vi "validate.vi"(8 "error in":errorcluster, 11 "Instrument configuration":refnum<class "Instrument configuration.lvclass">) -> (0 "error out":errorcluster, 3 "Instrument configuration out":refnum<class "Instrument configuration.lvclass">)   [LabVIEW 2025, in "Abstract Engine.lvlib" / "Instrument configuration.lvclass"]
doc: "Provides an interface for performing validation on a given configuration. Any children should define the behavior of this function to ensure that the configuration in memory can be used by the runtime class.Copyright 2017 National Instruments Corporation\n\nLicensed under the Apache License, Version 2.0 (the \"License\"); you may not use this file except in compliance with the License. You may obtain a copy of the License at http://www.apache.org/licenses/LICENSE-2.0\nUnless required by applicable law or agreed to in writing, software distributed under the License is distributed on an \"AS IS\" BASIS, WITHOUT WARRANTIES OR CONDITIONS OF ANY KIND, either express or implied. See the License for the specific language governing permissions and limitations under the License."
uses:
  Instrument configuration.lvclass
  Instrument configuration.lvclass/Instrument configuration.ctl
  Users/Public/Documents/Sandia National Labs/TSS Plugin/CEF.lvlibp
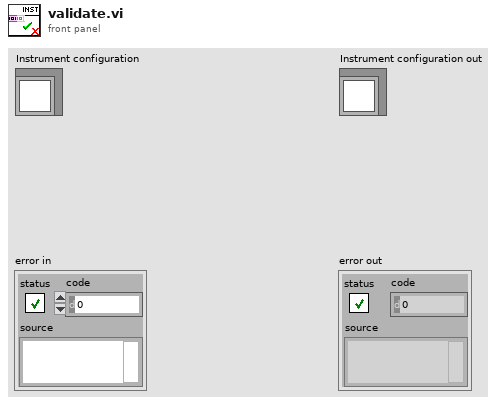
[diagram p1: front panel]
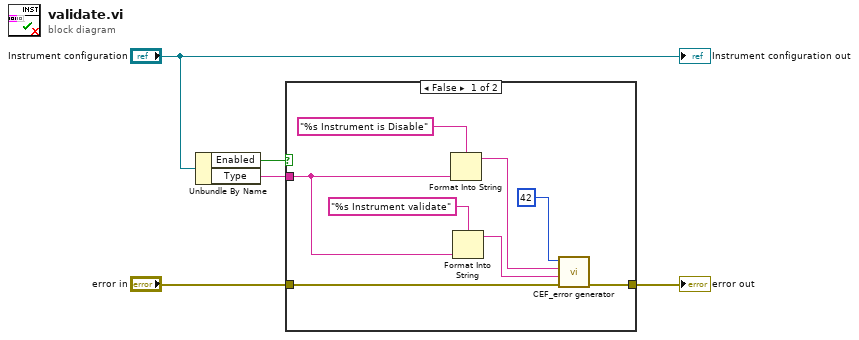
[diagram p0: block diagram]
diagram:
  n1 = Unbundle By Name("Instrument configuration") -> ("Enabled"=w2:bool, "Type"=w1:string)
  n2 = case shown="False" w2 {
    tunnel: "error in" -> [w13 w14]
    tunnel: [w11 w14] -> w4
    tunnel: w1 -> [w8 _]
    frame False {
      n3 = Format Into String(format string="%s Instrument is Disable" ("append error message"), w8) -> (resulting string=w9:string)  [unwired: 2 in, 1 out]
      n4 = Format Into String(format string="%s Instrument validate" ("source"), w8) -> (resulting string=w6:string)  [unwired: 2 in, 1 out]
      n5 = call "CEF_error generator.vi"("error in"=w13, "source"=w6, "append error message"=w9, "error code (0)"=42) -> ("error out"=w11:errorcluster)  [unwired: 5 in]
    }
    frame True {
    }
  }
  "error out" <- w4
  "Instrument configuration out" <- "Instrument configuration"
